vi "Acq_calibr.vi"(0 "Refnum in":refnum<k20>, 1 "refnum in":refnum<file>, 5 "Time to Acquire Block (ms)":i32, 7 "Block Size":u32, 9 "error out 3":errorcluster, 11 "error in (no error)":errorcluster, 12 "Inicio pasada 3":timestamp) -> (3 "refnum out 2":refnum<file>, 4 "Refnum out":refnum<k20>, 6 "Buffer Underflow 2":bool, 8 "error out 4":errorcluster, 10 "Buffer Overflow 2":bool, 15 "error out":errorcluster)   [LabVIEW 2015]
uses:
  <vilib>/rvi/interface/nirviMethod/nirviMethod.xnode
  FPGA Bitfiles/W&RDArabia_FPGATarget_FPGA8a2wsBIdirec_yJvL9yuTbZw.lvbitx
  <vilib>/rvi/errors/niLvFpgaMergeErrorWithErrorCode.vi
  <vilib>/rvi/interface/nirviReadWriteControl/nirviReadWriteControl.xnode
  <vilib>/FPGAPlugInAG/cRIO-9031/niLvFpga_ReadFifo_cRIO-9031.vi
  <vilib>/rvi/errors/niLvFpgaAdjustHostInterfaceError.vi
  <vilib>/FPGAPlugInAG/cRIO-9031/niLvFpga_StopFifo_cRIO-9031.vi
panel:
  out "Acquiring time":dbl
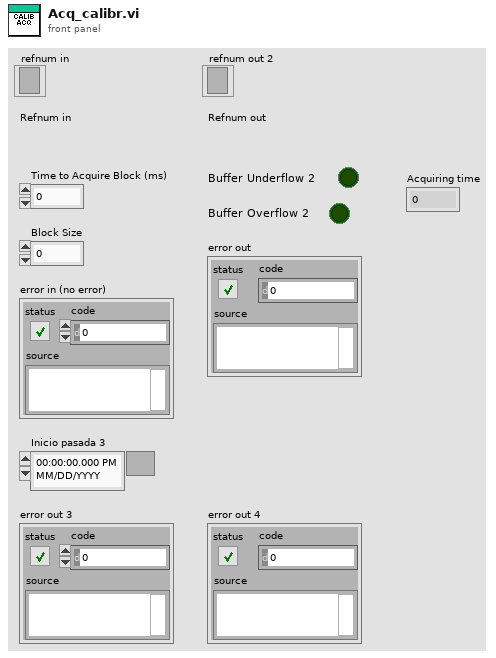
[diagram p1: front panel]
types:
  T1 = enum16{"big-endian, network order", "native, host order", "little-endian"}
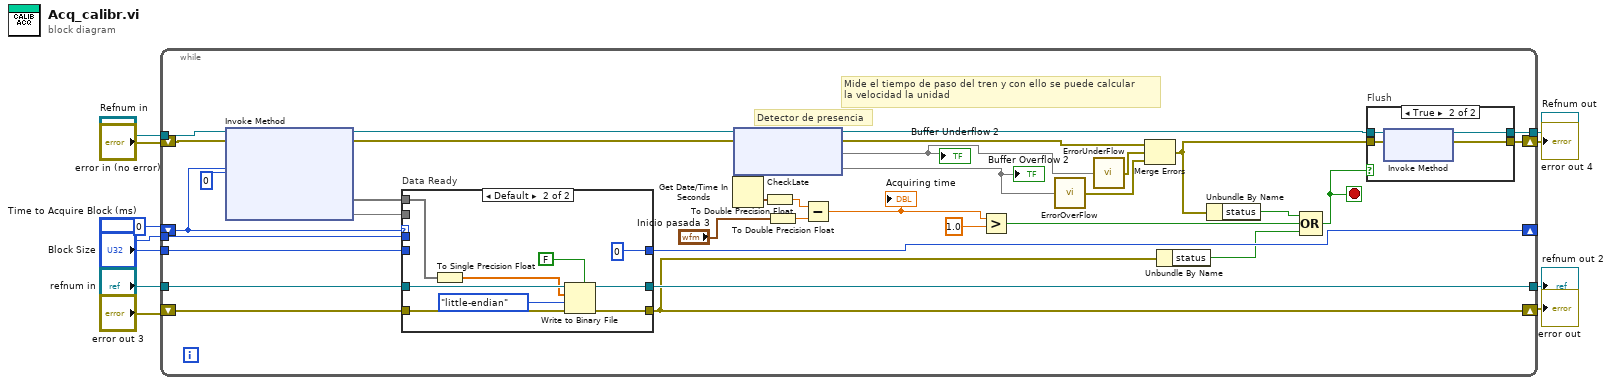
[diagram p0: block diagram]
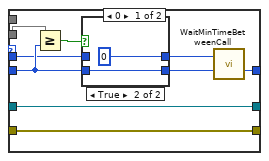
[diagram p2: hidden frame]
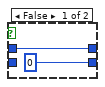
[diagram p3: hidden frame]
diagram:
  n1 = while "Data Acquisition" {
    tunnel: "Refnum in" -> [w36]
    shift-right: [w43] -> _
    shift-left: u32 0 ("t") -> [w39]
    tunnel: "Time to Acquire Block (ms)" -> [w44]
    tunnel: "Block Size" -> [w42]
    shift-right: [w45] -> w3
    shift-left: "error in (no error)" -> [w35]
    tunnel: [w40] -> w2
    tunnel: "refnum in" -> [w25]
    tunnel: [w26] -> w4
    shift-right: [w24] -> w11
    shift-left: "error out 3" -> [w33]
    stop <- w41 stop-if-true
    # "Detector de presencia"
    # "Mide el tiempo de paso del tren y con ello se puede calcular\nla velocidad la unidad"
    n2 = xnode "Invoke Method"("FPGA VI Reference In"=w36, "error in"=w35, "Number of Elements"=w39, "Timeout (ms)"=0) -> ("FPGA VI Reference Out"=w23:refnum<k20>, "error out"=w22:errorcluster, "Data"=w34:void[], "Elements Remaining"=w37)
    n3 = case "Data Ready" shown="Default" w39 {
      tunnel: w44 -> [w50 _]
      tunnel: [w49 u32 0 ("t")] -> w43
      tunnel: w42 -> [w51 _]
      tunnel: w37 -> [w48 _]
      tunnel: w34 -> [_ w61]
      tunnel: w33 -> [w47 w63]
      tunnel: [w47 w62] -> w24
      tunnel: w25 -> [w46 w60]
      tunnel: [w46 w59] -> w26
      frame 0 {
        n4 = Greater Or Equal?(x=w48, y=w51) -> (x >= y?=w52:bool)
        n5 = case shown="True" w52 {
          tunnel: [u32 0 ("Block Size") w56] -> w49
          tunnel: [w55 0 ("t")] -> w53
          tunnel: w50 -> [w55 _]
          tunnel: w51 -> [_ w56]
          frame False {
          }
          frame True {
          }
        }
        n6 = call "WaitMinTimeBetweenCall.vi"("Minimum ms between calls"=w53) -> ()  [unwired: 2 in]
      }
      frame Default {
        n7 = To Single Precision Float(number=w61) -> (single precision float=w58:sgl[])
        n8 = Write to Binary File(file (use dialog)=w60, data=w58, error in=w63, 5:FALSE ("prepend array or string size? (T)"), 9:T1."little-endian" ("byte order (0:big-endian, network order)")) -> (refnum out=w59:refnum<file>, error out=w62:errorcluster)  [unwired: 2 out]
      }
    }
    n9 = Get Date/Time In Seconds() -> (seconds since 1Jan1904=w20:timestamp)
    n10 = xnode ("CheckLate")("FPGA VI Reference In"=w23, "error in"=w22) -> ("FPGA VI Reference Out"=w16:refnum<k20>, "error out"=w31:errorcluster, "Buffer Underflow"=w13, "Buffer Overflow"=w12)
    "Buffer Underflow 2" <- w13
    "Buffer Overflow 2" <- w12
    n11 = To Double Precision Float(number=w20) -> (double precision float=w19:dbl)
    n12 = To Double Precision Float(number="Inicio pasada 3") -> (double precision float=w21:dbl)
    n13 = Subtract(x=w19, y=w21) -> (x-y=w28:dbl)
    "Acquiring time" <- w28
    n14 = Greater?(x=w28, y=1.0 ("Tiempo de adquisición")) -> (0:w18:bool)
    n15 = call "ErrorOverFlow.vi"("Buffer Overflow"=w12) -> ("error out"=w29:errorcluster)
    n16 = call "ErrorUnderFlow.vi"("Buffer Overflow"=w13) -> ("error out"=w30:errorcluster)
    n17 = Merge Errors(w31, w30, w29) -> (w17:errorcluster)
    n18 = Unbundle By Name(w24) -> ("status"=w27:bool)
    n19 = Unbundle By Name(w17) -> ("status"=w32:bool)
    n20 = Compound Arithmetic op=OR(w32, w18, w27) -> (w41:bool)
    n21 = case "Flush" shown="True" w41 {
      tunnel: w16 -> [w67 w72]
      tunnel: w17 -> [w68 w71]
      tunnel: [w68 w70] -> w45
      tunnel: [w67 w69] -> w40
      frame False {
      }
      frame True {
        n22 = xnode "Invoke Method"("FPGA VI Reference In"=w72, "error in"=w71) -> ("FPGA VI Reference Out"=w69:refnum<k20>, "error out"=w70:errorcluster)
      }
    }
  }
  "error out" <- w11
  "refnum out 2" <- w4
  "error out 4" <- w3
  "Refnum out" <- w2
